vi "File data.vi"(3 "error in":errorcluster, 5 "file path (use dialog)":path) -> (0 "error out":errorcluster, 2 "File data":string)   [LabVIEW 2018]
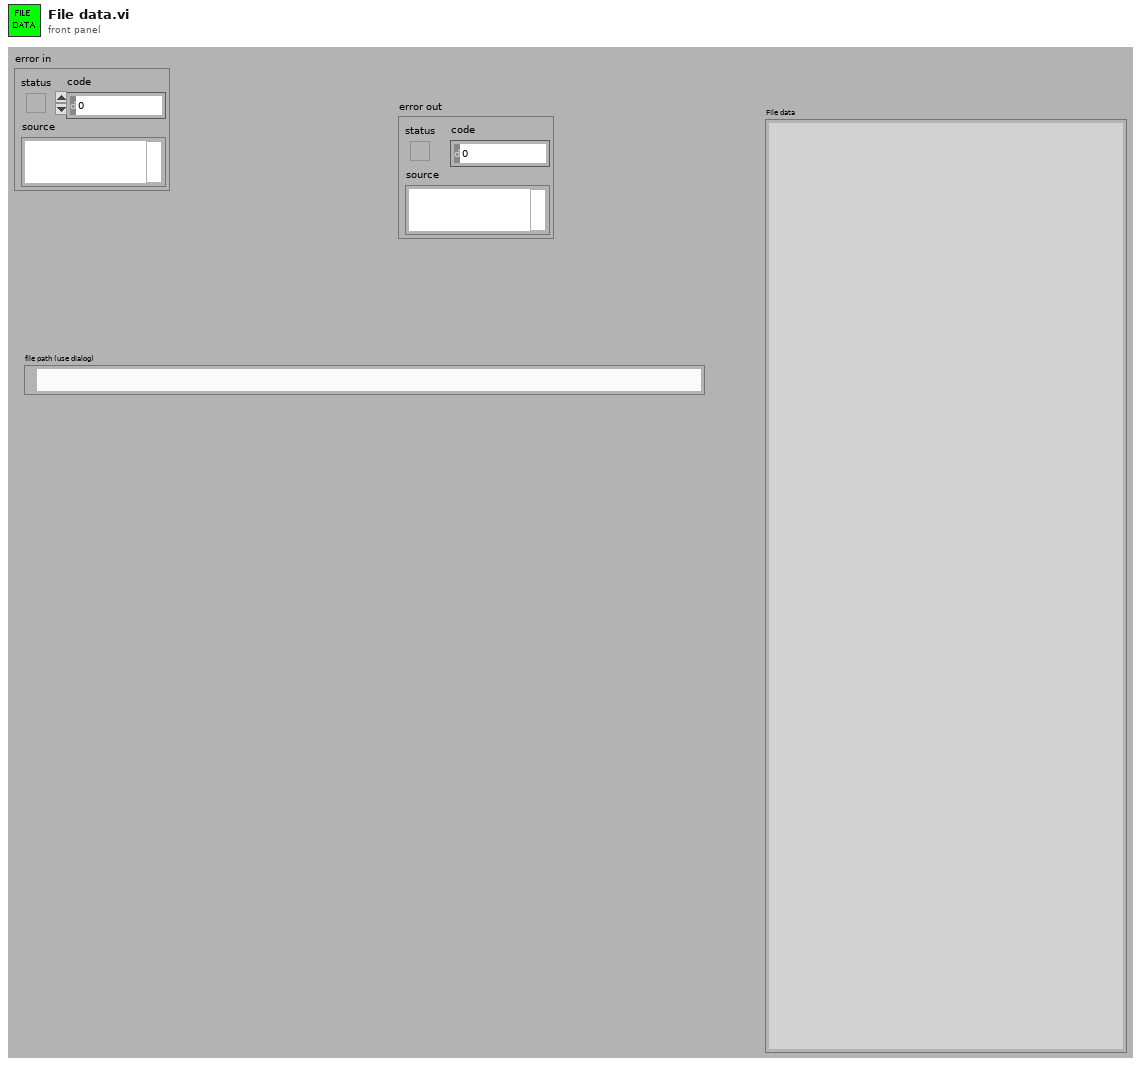
[diagram p1: front panel]
types:
  T1 = enum16{"open", "replace", "create", "open or create", "replace or create", "replace or create with confirmation"}
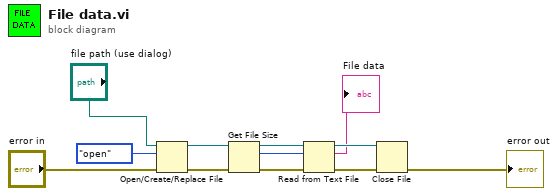
[diagram p0: block diagram]
diagram:
  n1 = Open/Create/Replace File(file path (use dialog)="file path (use dialog)", error in="error in", operation (0:open)=T1."open") -> (refnum out=w12:refnum<file>, error out=w11:errorcluster)  [unwired: 4 out]
  n2 = Get File Size(file=w12, error in=w11) -> (refnum out=w7:refnum<file>, size (in bytes)=w5:i64, 0:w6:errorcluster)
  n3 = Read from Text File(file (use dialog)=w7, count=w5, error in=w6) -> (refnum out=w4:refnum<file>, text=→"File data":string, error out=w3:errorcluster)  [unwired: 2 out]
  n4 = Close File(refnum=w4, error in=w3) -> (error out=→"error out":errorcluster)  [unwired: 1 out]
